vi "Execute Command.vi"(8 "error in (no error)":errorcluster, 10 "Command In":refnum<class "Command.lvclass">, 11 "Waiting in":refnum<class "Waiting.lvclass">) -> (0 "error out":errorcluster, 3 "Waiting out":refnum<class "Waiting.lvclass">)   [LabVIEW 2013, in "Command Processor.lvlib" / "Waiting.lvclass"]
uses:
  Waiting.lvclass
  Command/Command.lvclass
  Command Processor.lvclass
  <vilib>/ActorFramework/Actor/Actor.lvclass/Actor.ctl
  <vilib>/ActorFramework/Message Enqueuer/Message Enqueuer.lvclass/Message Enqueuer.ctl
  <vilib>/ActorFramework/Message Enqueuer/Init from Existing Queue.vi
  <vilib>/ActorFramework/Message Enqueuer/Enqueue.vi
  <vilib>/ActorFramework/Message Priority Queue/Priority Enqueue.vi
  <vilib>/ActorFramework/Message Enqueuer/Message Enqueuer.lvclass
  Command Processor Messages/Go To Executing Msg/Go To Executing Msg.lvclass
  <vilib>/ActorFramework/Actor/Actor.lvclass
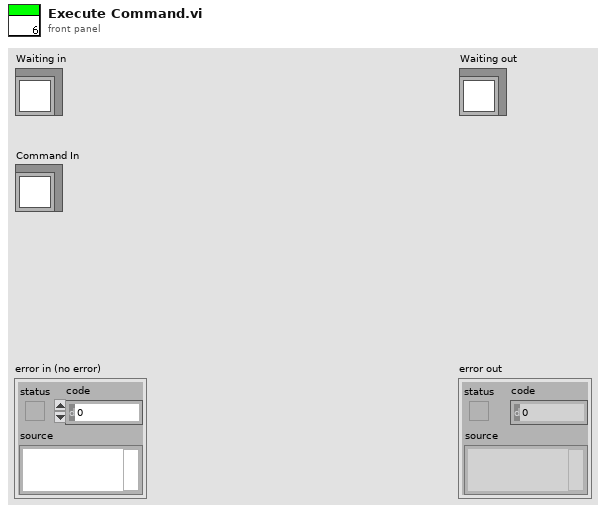
[diagram p1: front panel]
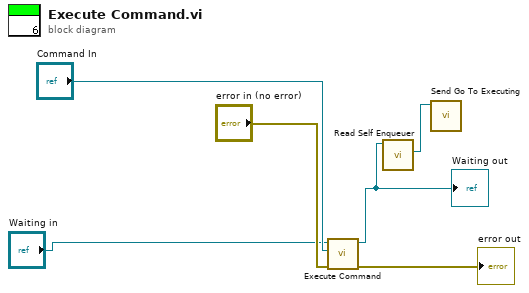
[diagram p0: block diagram]
diagram:
  n1 = call-parent "Execute Command.vi"("error in (no error)"="error in (no error)", "Command In"="Command In", "Command Processor in"="Waiting in") -> ("error out"=→"error out":errorcluster, "Command Processor out"=w2:refnum<class "Waiting.lvclass">)  [unwired: 7 in]
  "Waiting out" <- w2
  n2 = call <vilib>:"Read Self Enqueuer.vi"("Actor"=w2) -> ("Self Enqueuer"=w1:refnum<class "Message Enqueuer.lvclass">)  [unwired: 10 in]
  n3 = call "Send Go To Executing.vi"("Message Enqueuer"=w1) -> ()  [unwired: 9 in, 2 out]
